vi "test.vi"() -> ()   [LabVIEW 2022 SP3]
panel:
  out "Measurement":dbl
  in  "Function (0: DC Volts)":u16(ring) items=["DC Volts", "AC Volts", "AC+DC Volts", "DC Current", "AC Current", "AC+DC Current", "2-Wire Resistance", "Frequency", "Period", "Diode", "Continuity"]
  out "error out":errorcluster
  in  "error in (no error)":errorcluster
  in  "Instrument In":refnum<visa-resource-name>
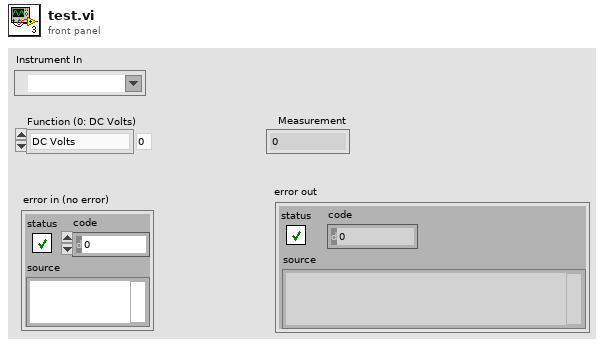
[diagram p1: front panel]
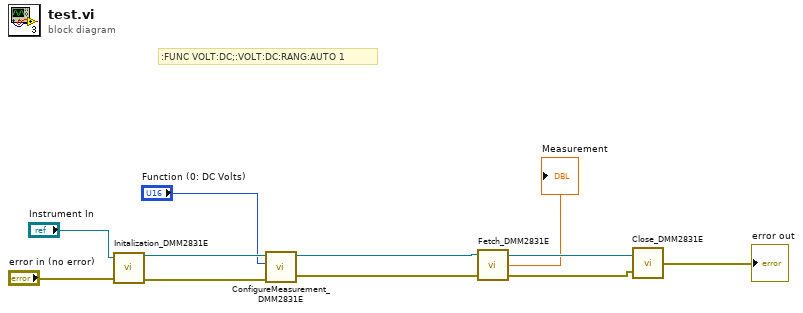
[diagram p0: block diagram]
diagram:
  # ":FUNC VOLT:DC;:VOLT:DC:RANG:AUTO 1"
  n1 = call "Initalization_DMM2831E.vi"("error in (no error)"="error in (no error)", "Instrument In"="Instrument In") -> ("error out"=w8:errorcluster, "Instrument Out"=w9:refnum<visa-resource-name>)  [unwired: 1 in]
  n2 = call "ConfigureMeasurement_DMM2831E.vi"("error in (no error)"=w8, "Function (0: DC Volts)"="Function (0: DC Volts)", "Instrument In"=w9) -> ("error out"=w5:errorcluster, "Instrument Out"=w6:refnum<visa-resource-name>)  [unwired: 3 in]
  n3 = call "Fetch_DMM2831E .vi"("error in (no error)"=w5, "VISA resource name"=w6) -> ("error out"=w3:errorcluster, "Measurement"=→"Measurement":dbl, "VISA resource name out"=w4:refnum<visa-resource-name>)  [unwired: 1 in]
  n4 = call "Close_DMM2831E .vi"("error in (no error)"=w3, "Instrument In"=w4) -> ("error out"=→"error out":errorcluster)
